vi "sub_Robot v0.vi"() -> ()   [LabVIEW 2017]
uses:
  <vilib>/Analysis/Matrix/Datatypes/RealMatrix.ctl
  Control/Force Torque Vector.ctl
  Control/State.ctl
  Control/Platform Vectors.ctl
  Control/Constants.ctl
  Control/Motor Position.ctl
  <vilib>/Analysis/baseanly.llb/A x Vector.vi
  <vilib>/DAQmx/read.llb/DAQmx Read (Analog 2D DBL NChan NSamp).vi
  <vilib>/Analysis/baseanly.llb/Mean (DBL).vi
  <vilib>/Analysis/baseanly.llb/Real A x B.vi
  <vilib>/Analysis/_algsub.llb/Vector Norm.vi
  <vilib>/Analysis/_algsub.llb/Real Vector Norm.vi
  <vilib>/Analysis/baseanly.llb/Outer Product.vi
  <vilib>/Analysis/baseanly.llb/Real Outer Product.vi
  <vilib>/robotics/Kinematics/Create Lie Group Matrix.vi
  <vilib>/Analysis/7linalg.llb/Create Special Real Matrix.vi
  <vilib>/Analysis/Matrix/Numeric/Multiply/Multiply.vi
  <vilib>/Analysis/Matrix/Numeric/Multiply/Multiply - RM,R.vi
  <vilib>/Analysis/Matrix/Numeric/Multiply/Multiply - R,RM.vi
  <vilib>/Analysis/Matrix/Numeric/Add/Add.vi
  <vilib>/Analysis/Matrix/Numeric/Add/Add - RM,RM.vi
  <vilib>/DAQmx/create/channels.llb/DAQmx Create Channel (AI-Voltage-Basic).vi
  <vilib>/DAQmx/configure/timing.llb/DAQmx Timing (Sample Clock).vi
  <vilib>/DAQmx/miscellaneous.llb/DAQmx Fill In Error Info.vi
  <vilib>/Analysis/3filter.llb/Butterworth Filter (DBL).vi
  <vilib>/Utility/inputDevices.llb/joystickAcquire.vi
  <vilib>/Analysis/NI_AALBase.lvlib
  <vilib>/robotics/Kinematics/NI_Kinematics.lvlib
  <vilib>/Analysis/NI_AALPro.lvlib
  <vilib>/Analysis/Matrix/NI_Matrix.lvlib
panel:
  in  "low cutoff freq: fl":dbl=0.1 format="%0.4f"
  in  "sampling freq: fs":dbl=100.0 format="%0.2f"
  in  "rate":dbl=1000.0 format="%#_13g"
  out "Motor Position":T1={"theta1"=1.8810837497796307, "theta2"=-0.7792215646198668, "theta3"=2.7030056815353944}
  in  "eta3":dbl=240.0
  in  "eta2":dbl=120.0
  in  "eta1":dbl
  out "dt":dbl=0.014741399998456473
  in  "gamma2":dbl=72.0
  in  "gamma1":dbl=90.0
  in  "alpha2":dbl=90.0
  in  "alpha1":dbl=90.0
  out "Constants":T2={"alpha1"=1.5707963267948966, "alpha2"=1.5707963267948966, "beta1"=0.9553166181245093, "beta2"=0.7460127831658564, "gamma1"=1.5707963267948966, "gamma2"=1.2566370614359172, "eta1"=0.0, "eta2"=2.0943951023931953, "eta3"=4.1887902047863905}
  out "Platform Vectors":T3={"v1"=[0.9518431395713998, -0.15246563731281282, 0.26598659193586577], "v2"=[0.43921969187034554, 0.8926089520236044, 0.10166278099993067], "v3"=[0.5741590303779587, 0.15523155866204005, -0.8038933828753619]}
  in  "radius":dbl=0.1
  in  "State":T4={"Inertia"=0.0, "Damping"=0.5, "RoM"=0.0}
  out "Waveform Chart":cluster{dbl, dbl, dbl}(graph)
  out "Force Torque Vector":T5
  in  "Calibration Matrix":T6=[[0.70287, 0.28046, -1.06379, -47.58271, -1.64459, 46.90249], [-0.12905, 55.12684, -1.23322, -27.09022, 0.94146, -27.44249], [69.23154, 1.17633, 67.18151, 0.05352, 69.14468, -0.82584], [0.02366, 0.38743, -1.10802, -0.19684, 1.1351, -0.20033], [1.26658, 0.02633, -0.60731, 0.32903, -0.6386, -0.32248], [0.02624, -0.70869, -0.00313, -0.69424, -0.02408, -0.68399]]
  in  "stop":bool
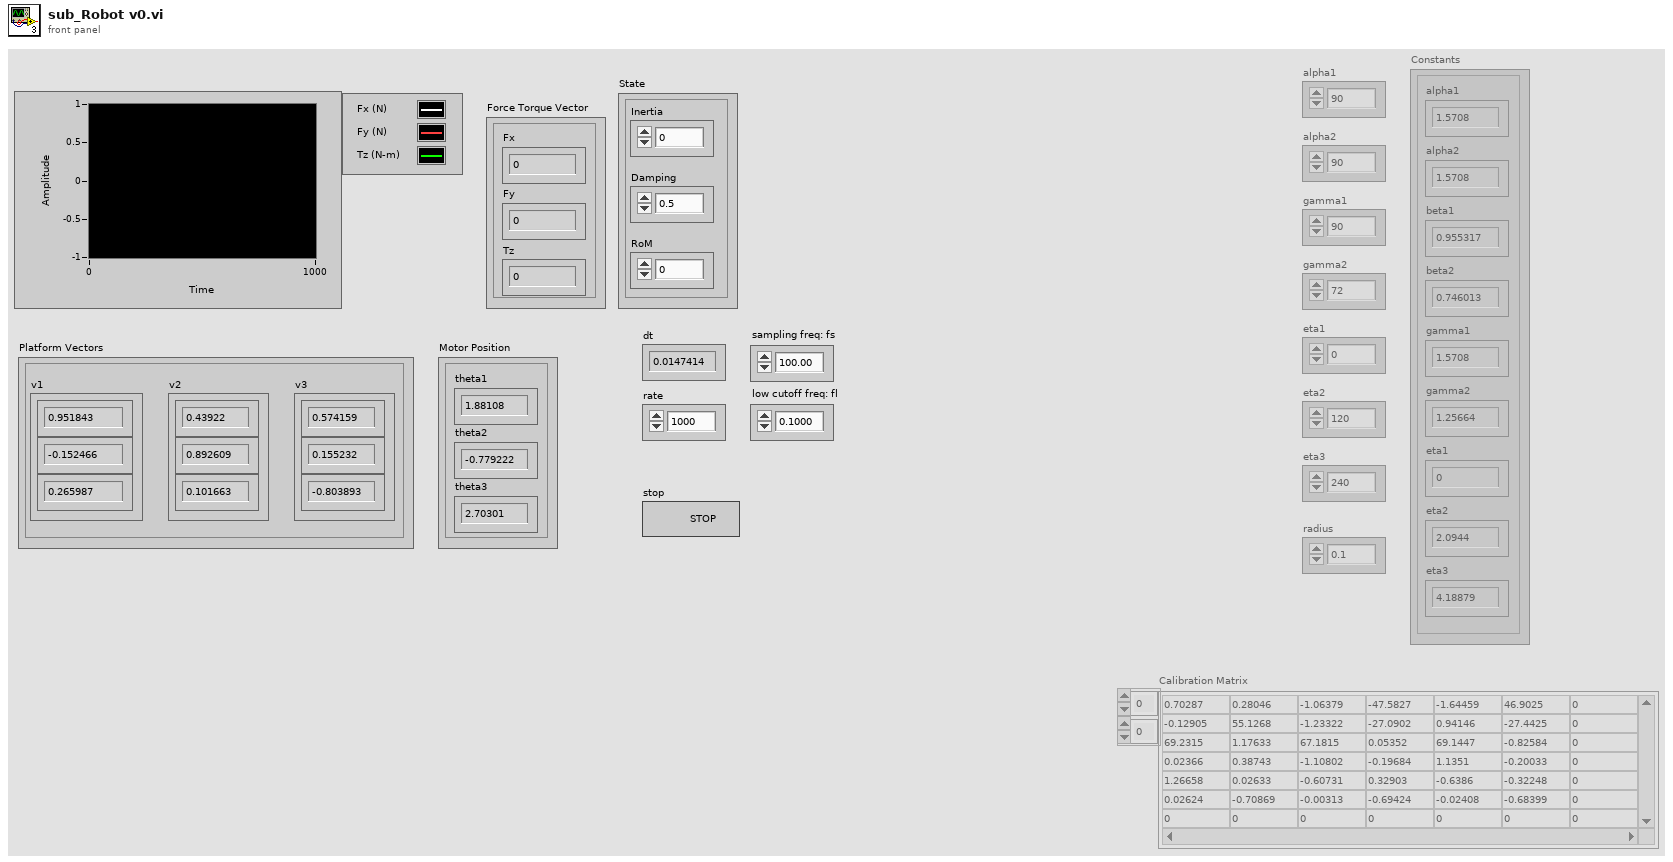
[diagram p1: front panel]
types:
  T1 = typedef "Motor Position.ctl" = cluster{"theta1":dbl, "theta2":dbl, "theta3":dbl}
  T2 = typedef "Constants.ctl" = cluster{"alpha1":dbl, "alpha2":dbl, "beta1":dbl, "beta2":dbl, "gamma1":dbl, "gamma2":dbl, "eta1":dbl, "eta2":dbl, "eta3":dbl}
  T3 = typedef "Platform Vectors.ctl" = cluster{"v1":dbl[], "v2":dbl[], "v3":dbl[]}
  T4 = typedef "State.ctl" = cluster{"Inertia":dbl, "Damping":dbl, "RoM":dbl}
  T5 = typedef "Force Torque Vector.ctl" = cluster{"Fx":dbl, "Fy":dbl, "Tz":dbl}
  T6 = typedef "NI_Matrix.lvlib/RealMatrix.ctl" = dbl[][]
  T7 = cluster{"X axis":i32, "Y axis":i32, "Z axis":i32, "X axis rotation":i32, "Y axis rotation":i32, "Z axis rotation":i32, "U axis":i32, "V axis":i32}
  T8 = cluster{"element":dbl, "element":dbl, "element":dbl}
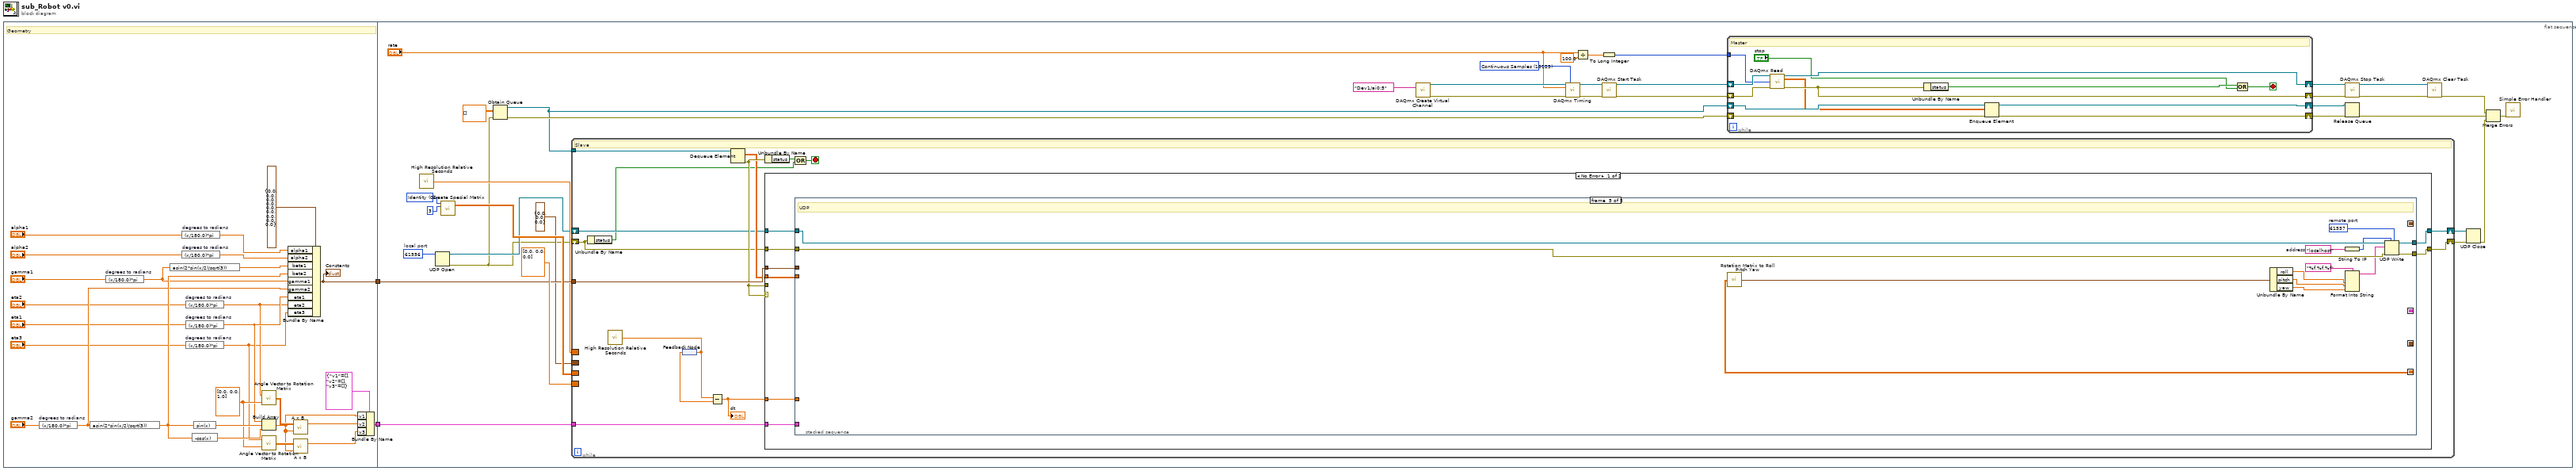
[diagram p0: block diagram]
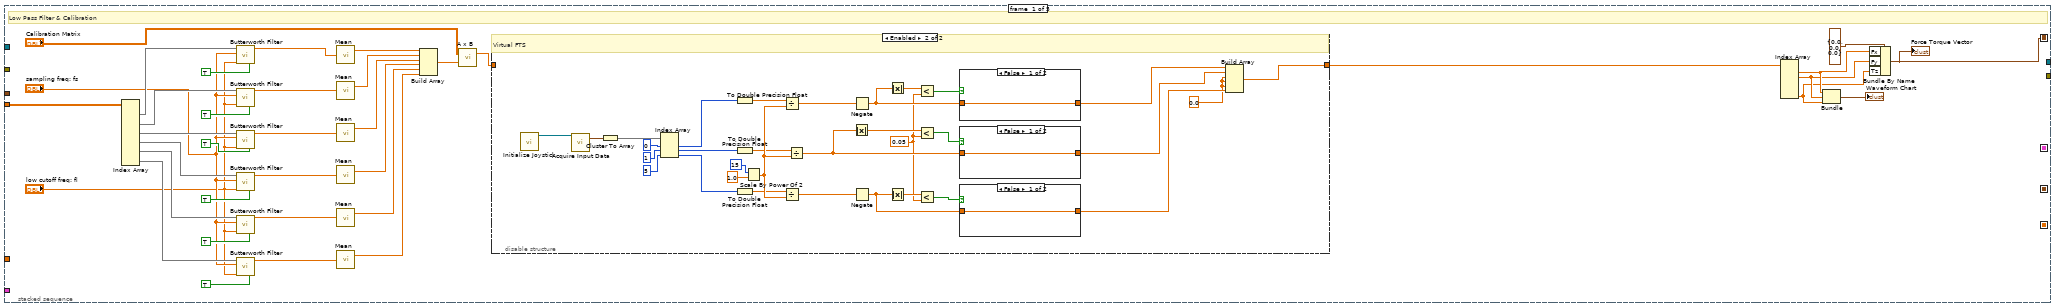
[diagram p2: hidden frame]
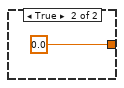
[diagram p4: hidden frame]
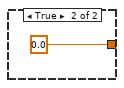
[diagram p5: hidden frame]
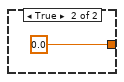
[diagram p6: hidden frame]
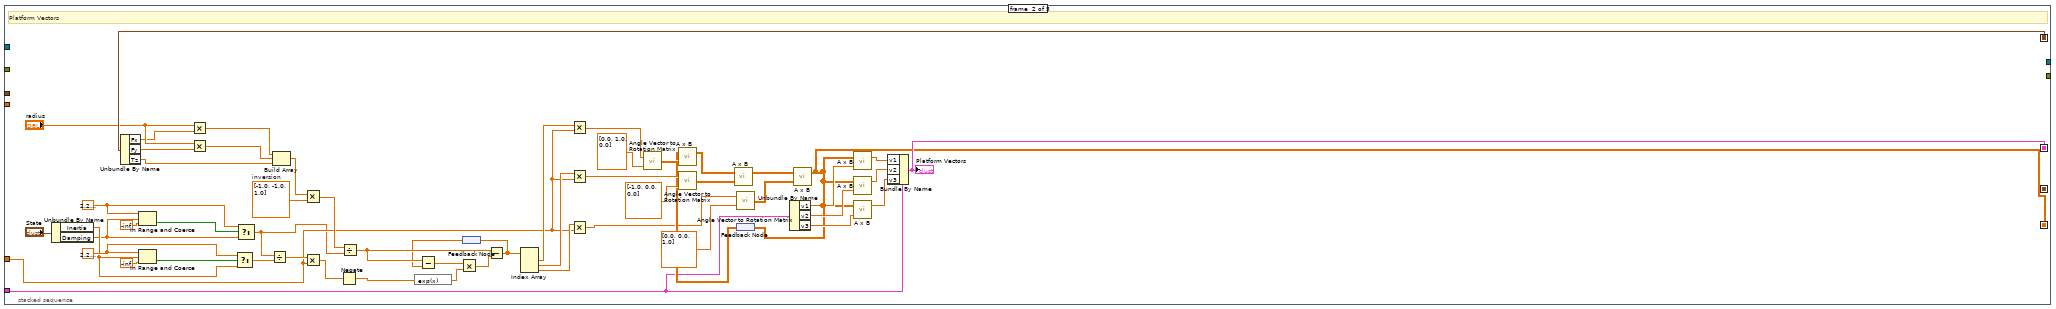
[diagram p7: hidden frame]
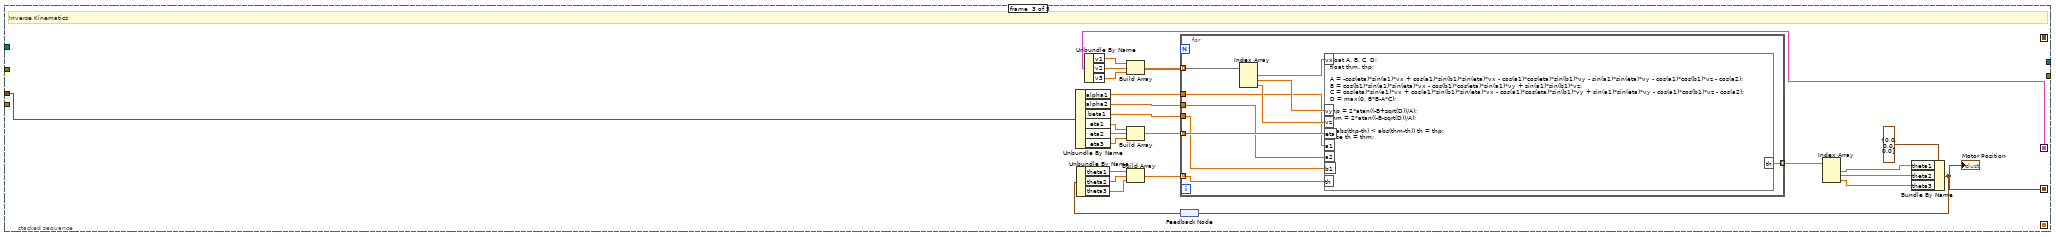
[diagram p8: hidden frame]
diagram:
  n1 = flat-sequence {
    tunnel: [w3] -> w2
    tunnel: [w5] -> w1
    tunnel: w2 -> [w46]
    tunnel: w1 -> [w45]
    frame #0 {
      w19 = dbl[] [0.0, 0.0, 1.0] ("vector")
      # "Geometry"
      n2 = expression code="(x/180.0)*pi" "degrees to radians"("gamma2") -> (w13:dbl)
      n3 = expression code="asin(2*sin(x/2)/sqrt(3))"(w13) -> (w15:dbl)
      n4 = expression code="(x/180.0)*pi" "degrees to radians"("gamma1") -> (w14:dbl)
      n5 = expression code="asin(2*sin(x/2)/sqrt(3))"(w14) -> (w26:dbl)
      n6 = expression code="(x/180.0)*pi" "degrees to radians"("alpha1") -> (w29:dbl)
      n7 = expression code="(x/180.0)*pi" "degrees to radians"("alpha2") -> (w27:dbl)
      n8 = expression code="(x/180.0)*pi" "degrees to radians"("eta2") -> (w8:dbl)
      n9 = expression code="(x/180.0)*pi" "degrees to radians"("eta1") -> (w9:dbl)
      n10 = expression code="(x/180.0)*pi" "degrees to radians"("eta3") -> (w7:dbl)
      n11 = expression code="-cos(x)"(w15) -> (w21:dbl)
      n12 = expression code="sin(x)"(w15) -> (w20:dbl)
      n13 = call <vilib>:"Angle Vector to Rotation Matrix.vi"("vector"=w19, "angle"=w8) -> ("rotation matrix"=w22:T6)
      n14 = Build Array(w9, w20, w21) -> (w18:dbl[])
      n15 = call <vilib>:"Angle Vector to Rotation Matrix.vi"("vector"=w19, "angle"=w7) -> ("rotation matrix"=w23:T6)
      n16 = Bundle By Name(cluster=T2 {"alpha1"=0.0, "alpha2"=0.0, "beta1"=0.0, "beta2"=0.0, "gamma1"=0.0, "gamma2"=0.0, "eta1"=0.0, "eta2"=0.0, "eta3"=0.0} ("Constants"), "alpha1"=w29, "alpha2"=w27, "beta1"=w26, "beta2"=w15, "gamma1"=w14, "gamma2"=w13, "eta1"=w9, "eta2"=w8, "eta3"=w7) -> (w5:T2)
      "Constants" <- w5
      n17 = call-poly <vilib>:"A x B.vi"("Vector"=w18, "A"=w22) -> ("A x Vector"=w17:dbl[])  [unwired: 1 out]
      n18 = call-poly <vilib>:"A x B.vi"("Vector"=w18, "A"=w23) -> ("A x Vector"=w16:dbl[])  [unwired: 1 out]
      n19 = Bundle By Name(cluster=T3 {"v1"=[], "v2"=[], "v3"=[]} ("Platform Vectors"), "v1"=w18, "v2"=w17, "v3"=w16) -> (w3:T3)
    }
    frame #1 {
      w36 = u16 61556  # local port
      w49 = 0 items=["Identity", "Diagonal", "Toeplitz", "Vandermonde", "Companion", "Hankel", "Hadamard", "Wilkinson", "Hilbert", "Inverse Hilbert", "Rosser", "Pascal"] ("matrix type")
      w57 = 10123 items=["Finite Samples"=10178, "Continuous Samples"=10123, "Hardware Timed Single Point"=12522] ("sample mode")
      n20 = call <vilib>:"High Resolution Relative Seconds.vi"() -> ("relative seconds"=w38:dbl)
      n21 = UDP Open(11:w36) -> (port=w34:refnum<k16>, 0:w31:errorcluster)  [unwired: 4 in, 1 out]
      n22 = call-poly <vilib>:"Create Special Matrix.vi"("matrix type"=w49, "matrix size"=3) -> ("Special Matrix"=w47:T6)  [unwired: 3 in, 1 out]
      n23 = Obtain Queue(element data type=dbl[][] [] ("data"), error in (no error)=w31) -> (queue out=w43:refnum<queue>, error out=w56:errorcluster)  [unwired: 3 in, 1 out]
      n24 = while {
        tunnel: w43 -> [w83]
        border: dbl[] [0.0, 0.0, 0.0] -> [_]
        border: w47 -> [_]
        tunnel: w45 -> [w81]
        border: T1 {"theta1"=0.0, "theta2"=0.0, "theta3"=0.0} ("Motor Position") -> [_]
        border: w38 -> [_]
        shift-right: [w77] -> w35
        shift-left: w31 -> [w74]
        tunnel: w46 -> [w82]
        shift-right: [w75] -> w33
        shift-left: w34 -> [w76]
        stop <- w71 stop-if-true
        # "Slave"
        n25 = Unbundle By Name(w74) -> ("status"=w72:bool)
        n26 = call <vilib>:"High Resolution Relative Seconds.vi"() -> ("relative seconds"=w70:dbl)
        n27 = feedback-in #1(w70) -> ()
        n28 = feedback #1() -> (w78:dbl)
        n29 = Subtract(x=w70, y=w78) -> (x-y=w69:dbl)
        "dt" <- w69
        n30 = Dequeue Element(queue=w83) -> (element=w79:dbl[][], error out=w80:errorcluster)  [unwired: 2 in, 2 out]
        n31 = Unbundle By Name(w80) -> ("status"=w73:bool)
        n32 = case shown="No Error" w80 {
          tunnel: w82 -> [w91 _]
          tunnel: w81 -> [w90 _]
          tunnel: w80 -> [_ _]
          tunnel: w79 -> [w89 _]
          tunnel: w69 -> [w88 _]
          tunnel: w74 -> [w87 w272]
          tunnel: w76 -> [w86 w271]
          tunnel: [w85 w271] -> w75
          tunnel: [w84 w272] -> w77
          frame No Error {
            n33 = stacked-sequence {
              seq-local: [w126 _ _ _ _] -> [_ w201 _ _ _]
              seq-local: [_ w184 _ _ _] -> [_ _ w225 _ _]
              seq-local: [_ _ w223 _ _] -> [_ _ _ _ _]
              seq-local: [_ w168 _ _ _] -> [_ _ _ _ w266]
              tunnel: w91 -> [_ w188 _ _ _]
              tunnel: w90 -> [_ _ w242 _ _]
              tunnel: w88 -> [_ w183 _ _ _]
              tunnel: w89 -> [w98 _ _ _ _]
              tunnel: w87 -> [_ _ _ _ w270]
              tunnel: w86 -> [_ _ _ _ w269]
              tunnel: [_ _ _ _ w268] -> w85
              tunnel: [_ _ _ _ w267] -> w84
              frame #0 {
                # "Low Pass Filter & Calibration"
                n34 = Index Array(array=w98) -> (element #1=w109:dbl[], element #2=w108:dbl[], element #3=w107:dbl[], element #4=w106:dbl[], element #5=w105:dbl[], element #6=w104:dbl[])  [unwired: 12 in]
                n35 = call-poly <vilib>:"Butterworth Filter.vi"("init/cont (init:F)"=TRUE, "low cutoff freq: fl"="low cutoff freq: fl", "sampling freq: fs"="sampling freq: fs", "X"=w109) -> ("Filtered X"=w110:dbl[])  [unwired: 4 in, 1 out]
                n36 = call-poly <vilib>:"Butterworth Filter.vi"("init/cont (init:F)"=TRUE, "low cutoff freq: fl"="low cutoff freq: fl", "sampling freq: fs"="sampling freq: fs", "X"=w108) -> ("Filtered X"=w112:dbl[])  [unwired: 4 in, 1 out]
                n37 = call-poly <vilib>:"Butterworth Filter.vi"("init/cont (init:F)"=TRUE, "low cutoff freq: fl"="low cutoff freq: fl", "sampling freq: fs"="sampling freq: fs", "X"=w107) -> ("Filtered X"=w114:dbl[])  [unwired: 4 in, 1 out]
                n38 = call-poly <vilib>:"Butterworth Filter.vi"("init/cont (init:F)"=TRUE, "low cutoff freq: fl"="low cutoff freq: fl", "sampling freq: fs"="sampling freq: fs", "X"=w106) -> ("Filtered X"=w115:dbl[])  [unwired: 4 in, 1 out]
                n39 = call-poly <vilib>:"Butterworth Filter.vi"("init/cont (init:F)"=TRUE, "low cutoff freq: fl"="low cutoff freq: fl", "sampling freq: fs"="sampling freq: fs", "X"=w105) -> ("Filtered X"=w116:dbl[])  [unwired: 4 in, 1 out]
                n40 = call-poly <vilib>:"Butterworth Filter.vi"("init/cont (init:F)"=TRUE, "low cutoff freq: fl"="low cutoff freq: fl", "sampling freq: fs"="sampling freq: fs", "X"=w104) -> ("Filtered X"=w120:dbl[])  [unwired: 4 in, 1 out]
                n41 = call-poly <vilib>:"Mean.vi"("X"=w110) -> ("mean"=w111:dbl)  [unwired: 1 out]
                n42 = call-poly <vilib>:"Mean.vi"("X"=w112) -> ("mean"=w113:dbl)  [unwired: 1 out]
                n43 = call-poly <vilib>:"Mean.vi"("X"=w114) -> ("mean"=w117:dbl)  [unwired: 1 out]
                n44 = call-poly <vilib>:"Mean.vi"("X"=w115) -> ("mean"=w118:dbl)  [unwired: 1 out]
                n45 = call-poly <vilib>:"Mean.vi"("X"=w116) -> ("mean"=w119:dbl)  [unwired: 1 out]
                n46 = call-poly <vilib>:"Mean.vi"("X"=w120) -> ("mean"=w121:dbl)  [unwired: 1 out]
                n47 = Build Array(w111, w113, w117, w118, w119, w121) -> (w96:dbl[])
                n48 = call-poly <vilib>:"A x B.vi"("Vector"=w96, "A"="Calibration Matrix") -> ("A x Vector"=w92:dbl[])  [unwired: 1 out]
                n49 = disable-structure shown="Enabled" {
                  disable-tunnel: [w129 w137] -> w93
                  disable-tunnel: w92 -> [w129 _]
                  frame Disabled {
                  }
                  frame Enabled {
                    w136 = 0.0 ("element")
                    w141 = 0.05 ("y")
                    # "Virtual FTS"
                    n50 = call <vilib>:"Initialize Joystick.vi"() -> ("device ID"=w154:refnum<k1>)  [unwired: 10 in, 1 out]
                    n51 = call-poly <vilib>:"Acquire Input Data.vi"("device ID"=w154) -> ("axis info"=w161:T7)  [unwired: 14 in, 4 out]
                    n52 = Cluster To Array(cluster=w161) -> (array=w157:i32[])
                    n53 = Index Array(array=w157, index #1=0 ("index"), index #2=1 ("index"), index #3=5 ("index")) -> (element #1=w135:i32, element #2=w133:i32, element #3=w131:i32)
                    n54 = To Double Precision Float(number=w135) -> (double precision float=w134:dbl)
                    n55 = To Double Precision Float(number=w133) -> (double precision float=w132:dbl)
                    n56 = To Double Precision Float(number=w131) -> (double precision float=w130:dbl)
                    n57 = Scale By Power Of 2(n=i16 15, x=1.0) -> (x*2^n=w149:dbl)
                    n58 = Divide(x=w134, y=w149) -> (x/y=w153:dbl)
                    n59 = Divide(x=w130, y=w149) -> (x/y=w142:dbl)
                    n60 = Divide(x=w132, y=w149) -> (x/y=w144:dbl)
                    n61 = Absolute Value(x=w144) -> (abs(x)=w151:dbl)
                    n62 = Negate(x=w153) -> (-x=w145:dbl)
                    n63 = Negate(x=w142) -> (-x=w143:dbl)
                    n64 = Absolute Value(x=w145) -> (abs(x)=w152:dbl)
                    n65 = Absolute Value(x=w143) -> (abs(x)=w150:dbl)
                    n66 = Less?(x=w152, y=w141) -> (x < y?=w148:bool)
                    n67 = Less?(x=w151, y=w141) -> (x < y?=w147:bool)
                    n68 = Less?(x=w150, y=w141) -> (x < y?=w146:bool)
                    n69 = case shown="False" w148 {
                      tunnel: [w166 0.0] -> w140
                      tunnel: w145 -> [w166 _]
                      frame False {
                      }
                      frame True {
                      }
                    }
                    n70 = case shown="False" w147 {
                      tunnel: [w164 0.0] -> w139
                      tunnel: w144 -> [w164 _]
                      frame False {
                      }
                      frame True {
                      }
                    }
                    n71 = case shown="False" w146 {
                      tunnel: [w162 0.0] -> w138
                      tunnel: w143 -> [w162 _]
                      frame False {
                      }
                      frame True {
                      }
                    }
                    n72 = Build Array(w140, w139, w136, w136, w136, w138) -> (w137:dbl[])
                  }
                }
                n73 = Index Array(array=w93) -> (element #1=w125:dbl, element #2=w124:dbl, element #6=w123:dbl)  [unwired: 6 in, 3 out]
                n74 = Bundle("element"=w125, "element"=w124, "element"=w123) -> (→"Waveform Chart":T8)  [unwired: 1 in]
                n75 = Bundle By Name(cluster=T5 {"Fx"=0.0, "Fy"=0.0, "Tz"=0.0} ("Force Torque Vector"), "Fx"=w125, "Fy"=w124, "Tz"=w123) -> (w126:T5)
                "Force Torque Vector" <- w126
              }
              frame #1 {
                w173 = 2.220446049250313e-16
                w176 = 2.220446049250313e-16
                w186 = dbl[] [-1.0, -1.0, 1.0]  # inversion
                # "Platform Vectors"
                n76 = Unbundle By Name("State") -> ("Inertia"=w175:dbl, "Damping"=w170:dbl)
                n77 = Unbundle By Name(w201) -> ("Fx"=w199:dbl, "Fy"=w198:dbl, "Tz"=w195:dbl)
                n78 = In Range and Coerce(upper limit=w173, x=w170, lower limit=-inf) -> (In Range?=w172:bool)  [unwired: 1 out]
                n79 = In Range and Coerce(upper limit=w176, x=w175, lower limit=-inf) -> (In Range?=w177:bool)  [unwired: 1 out]
                n80 = Multiply(x="radius", y=w199) -> (x*y=w197:dbl)
                n81 = Multiply(x="radius", y=w198) -> (x*y=w196:dbl)
                n82 = Select(t=w176, s=w177, f=w175) -> (s? t:f=w174:dbl)
                n83 = Select(t=w173, s=w172, f=w170) -> (s? t:f=w169:dbl)
                n84 = Divide(x=w169, y=w174) -> (x/y=w212:dbl)
                n85 = Build Array(w197, w196, w195) -> (w187:dbl[])
                n86 = Multiply(x=w187, y=w186) -> (x*y=w185:dbl[])
                n87 = Multiply(x=w212, y=w183) -> (x*y=w211:dbl)
                n88 = Negate(x=w211) -> (-x=w210:dbl)
                n89 = Divide(x=w185, y=w169) -> (x/y=w207:dbl[])
                n90 = expression code="exp(x)"(w210) -> (w208:dbl)
                n91 = feedback #2() -> (w193:dbl[])
                n92 = Subtract(x=w207, y=w193) -> (x-y=w209:dbl[])
                n93 = Multiply(x=w209, y=w208) -> (x*y=w206:dbl[])
                n94 = Subtract(x=w207, y=w206) -> (x-y=w194:dbl[])
                n95 = feedback-in #2(w194) -> ()
                n96 = Index Array(array=w194) -> (element #1=w204:dbl, element #2=w203:dbl, element #3=w205:dbl)  [unwired: 3 in]
                n97 = Multiply(x=w204, y=w183) -> (x*y=w222:dbl)
                n98 = Multiply(x=w203, y=w183) -> (x*y=w221:dbl)
                n99 = Multiply(x=w205, y=w183) -> (x*y=w182:dbl)
                n100 = call <vilib>:"Angle Vector to Rotation Matrix.vi"("vector"=dbl[] [0.0, 1.0, 0.0], "angle"=w222) -> ("rotation matrix"=w217:T6)
                n101 = call <vilib>:"Angle Vector to Rotation Matrix.vi"("vector"=dbl[] [-1.0, 0.0, 0.0], "angle"=w221) -> ("rotation matrix"=w215:T6)
                n102 = call <vilib>:"Angle Vector to Rotation Matrix.vi"("vector"=dbl[] [0.0, 0.0, 1.0], "angle"=w182) -> ("rotation matrix"=w213:T6)
                n103 = feedback #3() -> (w192:T6)
                n104 = call-poly <vilib>:"A x B.vi"("B"=w217, "A"=w192) -> ("A x B"=w216:T6)  [unwired: 1 out]
                n105 = call-poly <vilib>:"A x B.vi"("B"=w215, "A"=w216) -> ("A x B"=w214:T6)  [unwired: 1 out]
                n106 = Unbundle By Name(w188) -> ("v1"=w191:dbl[], "v2"=w190:dbl[], "v3"=w189:dbl[])
                n107 = call-poly <vilib>:"A x B.vi"("B"=w213, "A"=w214) -> ("A x B"=w168:T6)  [unwired: 1 out]
                n108 = feedback-in #3(w168) -> ()
                n109 = call-poly <vilib>:"A x B.vi"("Vector"=w191, "A"=w168) -> ("A x Vector"=w181:dbl[])  [unwired: 1 out]
                n110 = call-poly <vilib>:"A x B.vi"("Vector"=w190, "A"=w168) -> ("A x Vector"=w180:dbl[])  [unwired: 1 out]
                n111 = call-poly <vilib>:"A x B.vi"("Vector"=w189, "A"=w168) -> ("A x Vector"=w179:dbl[])  [unwired: 1 out]
                n112 = Bundle By Name(cluster=w188, "v1"=w181, "v2"=w180, "v3"=w179) -> (w184:T3)
                "Platform Vectors" <- w184
              }
              frame #2 {
                # "Inverse Kinematics"
                n113 = Unbundle By Name(w242) -> ("alpha1"=w237:dbl, "alpha2"=w236:dbl, "beta1"=w235:dbl, "eta1"=w241:dbl, "eta2"=w240:dbl, "eta3"=w239:dbl)
                n114 = Unbundle By Name(w225) -> ("v1"=w246:dbl[], "v2"=w245:dbl[], "v3"=w244:dbl[])
                n115 = Build Array(w246, w245, w244) -> (w243:dbl[][])
                n116 = Build Array(w241, w240, w239) -> (w238:dbl[])
                n117 = feedback #4() -> (w230:T1)
                n118 = Unbundle By Name(w230) -> ("theta1"=w229:dbl, "theta2"=w228:dbl, "theta3"=w227:dbl)
                n119 = Build Array(w229, w228, w227) -> (w226:dbl[])
                n120 = for {
                  tunnel: w243 -> [w256] mode=indexing
                  tunnel: w238 -> [w252] mode=indexing
                  tunnel: w237 -> [w251]
                  tunnel: w236 -> [w250]
                  tunnel: w235 -> [w249]
                  tunnel: [w248] -> w234 mode=indexing
                  tunnel: w226 -> [w247] mode=indexing
                  n121 = Index Array(array=w256) -> (element #1=w255:dbl, element #2=w254:dbl, element #3=w253:dbl)  [unwired: 3 in]
                  n122 = formula code="float A, B, C, D;\nfloat thm, thp;\n\nA = -cos(eta)*sin(a1)*vx + cos(a1)*sin(b1)*sin(eta)*vx - cos(a1)*cos(eta)*sin(b1)*vy - sin(a1)*sin(eta)*vy - cos(a1)*cos(b1)*vz - cos(a2);\nB = cos(b1)*sin(a1)*sin(eta)*vx - cos(b1)*cos(eta)*sin(a1)*vy + sin(a1)*sin(b1)*vz;\nC = cos(eta)*sin(a1)*vx + cos(a1)*sin(b1)*sin(eta)*vx - cos(a1)*cos(eta)*sin(b1)*vy + sin(a1)*sin(eta)*vy - cos(a1)*cos(b1)*vz - cos(a2);\nD = max(0, B*B-A*C);\n\nthp = 2*atan((-B+sqrt(D))/A); \nthm = 2*atan((-B-sqrt(D))/A); \n\nif(abs(thp-th) < abs(thm-th)) th = thp;\nelse th = thm;"("vx"=w255, "vy"=w254, "vz"=w253, "eta"=w252, "a1"=w251, "b1"=w249, "a2"=w250, "th"=w247) -> ("th"=w248:dbl)
                }
                n123 = Index Array(array=w234) -> (element #1=w233:dbl, element #2=w232:dbl, element #3=w231:dbl)  [unwired: 3 in]
                n124 = Bundle By Name(cluster=T1 {"theta1"=0.0, "theta2"=0.0, "theta3"=0.0} ("Motor Position"), "theta1"=w233, "theta2"=w232, "theta3"=w231) -> (w223:T1)
                "Motor Position" <- w223
                n125 = feedback-in #4(w223) -> ()
              }
              frame #3 {
                # "myRIO"
              }
              frame #4 {
                w259 = u16 61557  # remote port
                w260 = "localhost"  # address
                # "UDP"
                n126 = call <vilib>:"Rotation Matrix to Roll Pitch Yaw.vi"("rotation matrix"=w266) -> ("angles"=w265:cluster{"roll":dbl, "pitch":dbl, "yaw":dbl})
                n127 = Unbundle By Name(w265) -> ("roll"=w264:dbl, "pitch"=w263:dbl, "yaw"=w262:dbl)
                n128 = String To IP(1:w260) -> (0:w258:u32)
                n129 = Format Into String(format string="%f,%f,%f", w264, w263, w262) -> (resulting string=w257:string)  [unwired: 2 in, 1 out]
                n130 = UDP Write(address=w258, port or service name=w259, connection ID=w269, data in=w257, 8:w270) -> (error out=w267:errorcluster, 3:w268:refnum<k16>)  [unwired: 1 in]
              }
            }
          }
          frame Error {
          }
        }
        n131 = Compound Arithmetic op=OR(w73, w72) -> (w71:bool)
      }
      n132 = call-poly <vilib>:"DAQmx Create Virtual Channel.vi"("physical channels"=tag "Dev1/ai0:5") -> ("task out"=w67:refnum<k21>, "error out"=w66:errorcluster)  [unwired: 13 in]
      n133 = call-poly <vilib>:"DAQmx Timing.vi"("task/channels in"=w67, "sample mode"=w57, "rate"="rate", "error in"=w66) -> ("task out"=w64:refnum<k21>, "error out"=w65:errorcluster)  [unwired: 10 in]
      n134 = Divide(x="rate", y=100.0) -> (x/y=w37:dbl)
      n135 = To Long Integer(number=w37) -> (32bit integer=w40:i32)
      n136 = call <vilib>:"DAQmx Start Task.vi"("task/channels in"=w64, "error in"=w65) -> ("task out"=w63:refnum<k21>, "error out"=w60:errorcluster)  [unwired: 12 in]
      n137 = while {
        shift-right: [w280] -> w53
        shift-left: w43 -> [w281]
        shift-right: [w277] -> w52
        shift-left: w56 -> [w279]
        shift-right: [w284] -> w62
        shift-left: w63 -> [w285]
        shift-right: [w282] -> w59
        shift-left: w60 -> [w283]
        tunnel: w40 -> [w273]
        stop <- w276 stop-if-true
        # "Master"
        n138 = call-poly <vilib>:"DAQmx Read.vi"("task/channels in"=w285, "number of samples per channel"=w273, "error in"=w283) -> ("task out"=w284:refnum<k21>, "data"=w274:dbl[][], "error out"=w282:errorcluster)  [unwired: 10 in]
        n139 = Unbundle By Name(w282) -> ("status"=w278:bool)
        n140 = Enqueue Element(queue=w281, element=w274, error in (no error)=w279) -> (queue out=w280:refnum<queue>, error out=w277:errorcluster)  [unwired: 1 in, 1 out]
        n141 = Compound Arithmetic op=OR(w278, "stop") -> (w276:bool)
      }
      n142 = call <vilib>:"DAQmx Stop Task.vi"("task/channels in"=w62, "error in"=w59) -> ("task out"=w61:refnum<k21>, "error out"=w58:errorcluster)  [unwired: 12 in]
      n143 = Release Queue(queue=w53, error in (no error)=w52) -> (error out=w51:errorcluster)  [unwired: 1 in, 2 out]
      n144 = call <vilib>:"DAQmx Clear Task.vi"("task in"=w61, "error in"=w58) -> ("error out"=w54:errorcluster)  [unwired: 13 in]
      n145 = UDP Close(connection ID=w33, 8:w35) -> (error out=w32:errorcluster)  [unwired: 1 out]
      n146 = Merge Errors(w54, w51, w32) -> (w55:errorcluster)
      n147 = call <vilib>:"Simple Error Handler.vi"("error in (no error)"=w55) -> ()  [unwired: 4 in, 5 out]
    }
  }
